vi "POST Multipart.vi"(6 "timeout (10000)":i32=10000, 7 "output file":path=path "", 8 "error in (no error)":errorcluster, 9 "data":T1[](array[typedef]), 10 "url":string, 11 "HTTP Client Advanced in":refnum<class "HTTP Client Advanced.lvclass">) -> (0 "error out":errorcluster, 1 "body":string, 2 "headers":string, 3 "HTTP Client Advanced out":refnum<class "HTTP Client Advanced.lvclass">)   [LabVIEW 2021, in "HTTP Client Advanced.lvclass"]
uses:
  HTTP Client Advanced.lvclass
  <vilib>/httpClient/MultipartData.ctl
  HTTP Client Advanced.lvclass/HTTP Client Advanced.ctl
  <vilib>/NI/Advanced HTTP Client/Session.lvclass
  <vilib>/httpClient/LabVIEWHTTPClient.lvlib
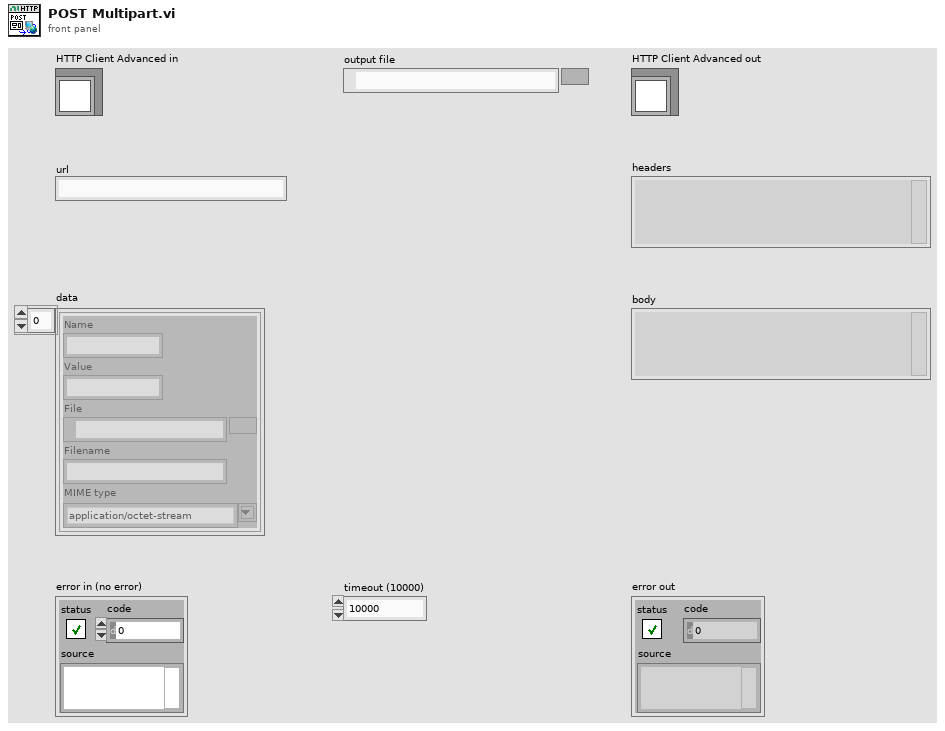
[diagram p1: front panel]
types:
  T1 = typedef "LabVIEWHTTPClient.lvlib/MultipartData.ctl" = cluster{"Name":string, "Value":string, "File":path, "Filename":string, "MIME type":string}
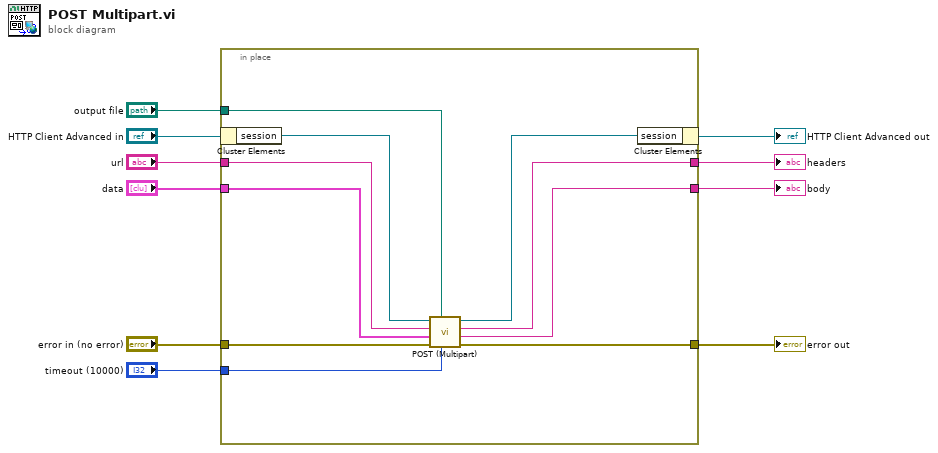
[diagram p0: block diagram]
diagram:
  n1 = in-place {
    in-place-border: "error in (no error)" -> [w20]
    in-place-border: [w19] -> w8
    in-place-border: "output file" -> [w16]
    in-place-border: "url" -> [w15]
    in-place-border: "data" -> [w14]
    in-place-border: [w13] -> w3
    in-place-border: [w12] -> w2
    in-place-border: "timeout (10000)" -> [w11]
    n2 = in-place-cluster #1("HTTP Client Advanced in") -> ("session"=w18:refnum<class "Session.lvclass">)
    n3 = call <vilib>:"POST (Multipart).vi"("timeout"=w11, "output file"=w16, "error in"=w20, "data"=w14, "url"=w15, "session in"=w18) -> ("error out"=w19:errorcluster, "body"=w12:string, "headers"=w13:string, "session out"=w17:refnum<class "Session.lvclass">)  [unwired: 1 in, 1 out]
    n4 = in-place-cluster #1("session"=w17) -> (→"HTTP Client Advanced out":refnum<class "HTTP Client Advanced.lvclass">)
  }
  "error out" <- w8
  "headers" <- w3
  "body" <- w2
